vi "SetUp.vi"(8 "error in (no error)":errorcluster, 11 "AjustesPrevios in":refnum<class "AjustesPrevios.lvclass">) -> (0 "error out":errorcluster, 3 "AjustesPrevios out":refnum<class "AjustesPrevios.lvclass">)   [LabVIEW 2019, in "AjustesPrevios.lvclass"]
uses:
  AjustesPrevios.lvclass
  Instrumento/Pistofono/Pistofono.lvclass
  D:/REPO/GitHub/procal/Instrumento/Instrumento/Instrumento.lvclass
  Instrumento/CNT90/CNT90.lvclass
  AjustesPrevios.lvclass/AjustesPrevios.ctl
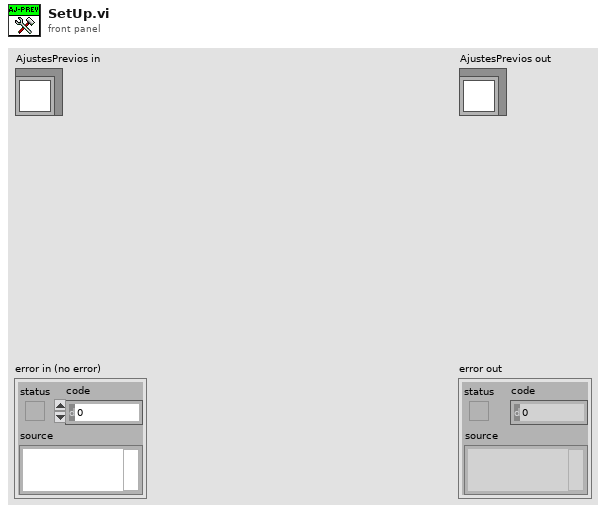
[diagram p1: front panel]
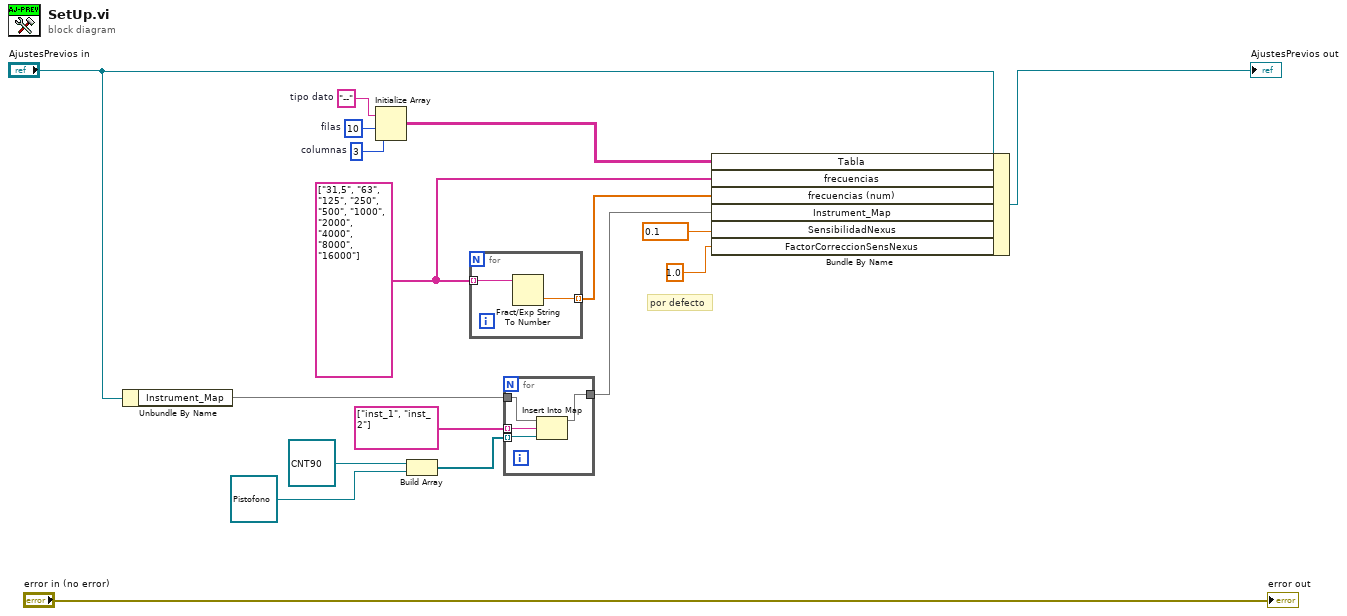
[diagram p0: block diagram]
diagram:
  w1 = 0.1 items=["10m"=0.01, "31,6m"=0.0316, "100m"=0.1, "316m"=0.316, "1"=1.0] ("Sensibilidad")
  w11 = string[] ["31,5", "63", "125", "250", "500", "1000", "2000", "4000", "8000", "16000"] ("subarray")
  w15 = 3  # columnas
  w16 = 10  # filas
  w14 = "--"  # tipo dato
  # "por defecto"
  n1 = Unbundle By Name("AjustesPrevios in") -> ("Instrument_Map"=w4:map{string, refnum<class "Instrumento.lvclass">})
  n2 = Initialize Array(w14, w16, w15) -> (w13:string[][])
  n3 = Build Array(refnum<class "CNT90.lvclass"> refnum ("CNT90.lvclass"), refnum<class "Pistofono.lvclass"> refnum ("Pistofono.lvclass")) -> (w6:refnum<class "Instrumento.lvclass">[])
  n4 = for {
    tunnel: w11 -> [w19] mode=indexing
    tunnel: [w18] -> w10 mode=indexing
    n5 = Fract/Exp String To Number(string=w19) -> (number=w18:dbl)  [unwired: 3 in, 1 out]
  }
  n6 = for {
    tunnel: w6 -> [w22] mode=indexing
    tunnel: string[] ["inst_1", "inst_2"] ("key") -> [w23] mode=indexing
    tunnel: w4 -> [w21]
    tunnel: [w20] -> w3
    n7 = Insert Into Map(map in=w21, key=w23, value=w22) -> (map out=w20:map{string, refnum<class "Instrumento.lvclass">})  [unwired: 2 out]
  }
  n8 = Bundle By Name(cluster="AjustesPrevios in", "Tabla"=w13, "frecuencias"=w11, "frecuencias (num)"=w10, "Instrument_Map"=w3, "SensibilidadNexus"=w1, "FactorCorreccionSensNexus"=1.0 ("igualacion_de_patrones.FactorCorreccionSensNexus")) -> (→"AjustesPrevios out":refnum<class "AjustesPrevios.lvclass">)
  "error out" <- "error in (no error)"
